vi "Registration.vi"() -> ()   [LabVIEW 2015]
uses:
  <vilib>/Analysis/Matrix/Datatypes/RealMatrix.ctl
  <vilib>/Analysis/Matrix/NI_Matrix.lvlib
panel:
  out "Array":dbl[](array[numeric])
  in  "Robot TCP Pose 2":T1
  in  "Selected tool":string(combo)
  out "Connected":bool
  in  "?":bool
  in  "Path to robot XML file":path
  in  "Ref System Pose":T1
  in  "Robot TCP Pose":T1
  in  "Grab current robot pose":bool
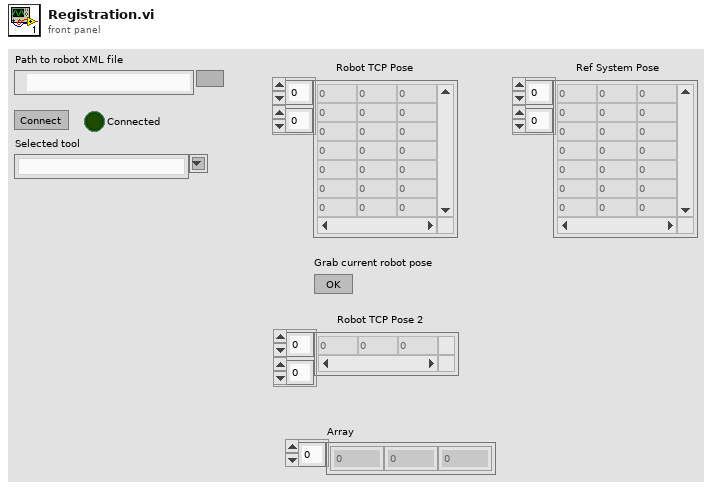
[diagram p1: front panel]
types:
  T1 = typedef "NI_Matrix.lvlib/RealMatrix.ctl" = dbl[][]
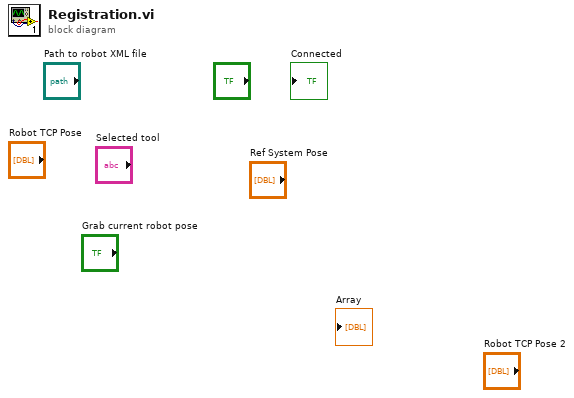
[diagram p0: block diagram]
diagram:
